vi "Bank - Semaphore.vi"() -> ()   [LabVIEW 2014]
doc: "This VI simulates the transactions that occur in a bank and demonstrates race conditions.\n\nRun the VI, and attempt a simultaneous transaction and notice that either the withdrawal or deposit is lost. Try to find and solve the problem."
panel:
  out "Balance":dbl
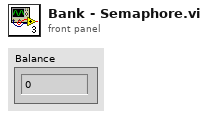
[diagram p1: front panel]
types:
  T1 = typedef "Account Info.ctl" = cluster{"Bank Rendezvous":T2, "Withdrawal Queue":refnum<queue>, "Deposit Queue":refnum<queue>}
  T2 = typedef "Rendezvous RefNum" = refnum<k1>
  T3 = typedef "Semaphore RefNum" = refnum<k1>
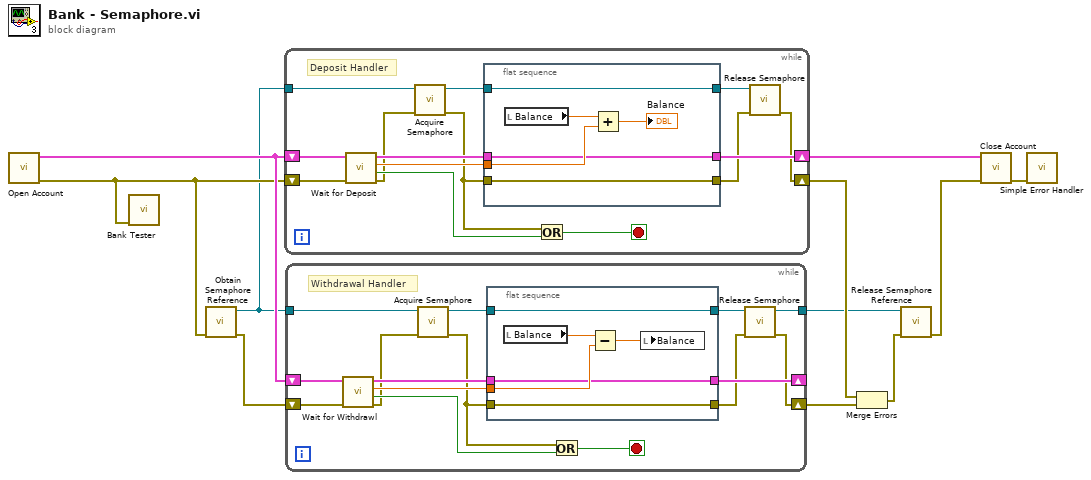
[diagram p0: block diagram]
diagram:
  n1 = call "Open Account.vi"() -> ("error out"=w6:errorcluster, "Account info"=w11:T1)  [unwired: 10 in]
  n2 = call "Bank Tester.vi"("error in"=w6) -> ()  [unwired: 10 in, 1 out]
  n3 = call <vilib>:"Obtain Semaphore Reference.vi"("error in (no error)"=w6) -> ("error out"=w5:errorcluster, "semaphore"=w1:T3)  [unwired: 4 in, 1 out]
  n4 = while {
    shift-right: [w21] -> w8
    shift-left: w11 -> [w24]
    shift-right: [w15] -> w10
    shift-left: w6 -> [w23]
    tunnel: w1 -> [w14]
    stop <- w19 stop-if-true
    # "Deposit Handler"
    n5 = call "Wait for Deposit.vi"("error in"=w23, "Account info"=w24) -> ("error out"=w18:errorcluster, "Stop?"=w20:bool, "Deposit Amount"=w25:dbl, "Account info out"=w22:T1)  [unwired: 6 in]
    n6 = call <vilib>:"Acquire Semaphore.vi"("error in (no error)"=w18, "semaphore"=w14) -> ("error out"=w17:errorcluster, "semaphore out"=w13:T3)  [unwired: 3 in, 1 out]
    n7 = flat-sequence {
      tunnel: w25 -> [w31]
      tunnel: [w28] -> w21
      tunnel: w22 -> [w28]
      tunnel: w17 -> [w27]
      tunnel: [w27] -> w16
      tunnel: w13 -> [w26]
      tunnel: [w26] -> w12
      frame #0 {
        n8 = local read "Balance"() -> (w29:dbl)
        n9 = Add(x=w29, y=w31) -> (x+y=→"Balance":dbl)
      }
    }
    n10 = Or(x=w17, y=w20) -> (x .or. y?=w19:bool)
    n11 = call <vilib>:"Release Semaphore.vi"("error in (no error)"=w16, "semaphore"=w12) -> ("error out"=w15:errorcluster)  [unwired: 4 in, 1 out]
  }
  n12 = while {
    shift-right: [w42] -> _
    shift-left: w11 -> [w45]
    shift-right: [w32] -> w9
    shift-left: w5 -> [w44]
    tunnel: w1 -> [w39]
    tunnel: [w36] -> w2
    stop <- w40 stop-if-true
    # "Withdrawal Handler"
    n13 = call "Wait for Withdrawl.vi"("error in"=w44, "Account info"=w45) -> ("error out"=w35:errorcluster, "Stop?"=w41:bool, "Withdrawal Amount"=w46:dbl, "Account info out"=w43:T1)  [unwired: 6 in]
    n14 = call <vilib>:"Acquire Semaphore.vi"("error in (no error)"=w35, "semaphore"=w39) -> ("error out"=w34:errorcluster, "semaphore out"=w38:T3)  [unwired: 3 in, 1 out]
    n15 = flat-sequence {
      tunnel: w46 -> [w50]
      tunnel: w43 -> [w49]
      tunnel: w34 -> [w48]
      tunnel: [w49] -> w42
      tunnel: [w48] -> w33
      tunnel: w38 -> [w47]
      tunnel: [w47] -> w37
      frame #0 {
        n16 = local read "Balance"() -> (w51:dbl)
        n17 = Subtract(x=w51, y=w50) -> (x-y=w52:dbl)
        n18 = local write "Balance"(w52) -> ()
      }
    }
    n19 = Or(x=w34, y=w41) -> (x .or. y?=w40:bool)
    n20 = call <vilib>:"Release Semaphore.vi"("error in (no error)"=w33, "semaphore"=w37) -> ("error out"=w32:errorcluster, "semaphore out"=w36:T3)  [unwired: 4 in]
  }
  n21 = Merge Errors(w10, w9) -> (w4:errorcluster)
  n22 = call <vilib>:"Release Semaphore Reference.vi"("error in (no error)"=w4, "semaphore"=w2) -> ("error out"=w3:errorcluster)  [unwired: 8 in, 1 out]
  n23 = call "Close Account.vi"("error in"=w3, "Account info"=w8) -> ("error out"=w7:errorcluster)  [unwired: 9 in]
  n24 = call <vilib>:"Simple Error Handler.vi"("error in (no error)"=w7) -> ()  [unwired: 4 in, 5 out]
